vi "OAT Order Power Spectrum (1 Channel).vi"(0 "even-angle signal":cluster{"r0":dbl, "dr":dbl, "Y":dbl[]}={"r0"=0.0, "dr"=1.0, "Y"=[]} {"r0" format="%.2p"; "dr" format="%.2p"; "Y" format="%.2f"}, 1 "dB on? (T)":bool=TRUE, 5 "even-angle channel info":T1={"channel name"="", "description"="", " channel info"={"sensor sensitivity"=1000.0, "engineering units"=1, "dB reference"=1.0, "custom label"="EU", "weighting filter"=0, "pregain"=0.0}} {"channel info"."pregain" format="%.2f"; "channel info"."weighting filter" items=["Linear", "A-weighting", "B-weighting", "C-weighting", "ITU-R 468-4", "Dolby", "CCITT", "C-message", "Wb", "Wc", "Wd", "We", "Wf", "Wh", "Wj", "Wk", "Wm", "AES17 20 kHz lowpass", "AES17 40 kHz lowpass", "AES17 20 kHz highpass", "AES17 40 kHz highpass"]; "channel info"."dB reference" format="%^.1e"; "channel info"."engineering units" items=["custom..."=0, "V"=1, "A"=21, "C"=30, "pC"=31, "s"=32, "-"=29, "Pa"=2, "N"=20, "g"=3, "m/s^2"=4, "m/s"=5, "m"=6, "mm/s"=12, "mm"=13, "micron/s"=14, "micron"=15, "in/s^2"=7, "in/s"=8, "in"=9, "mil/s"=10, "mil"=11, "rad/s^2"=16, "rad/s"=17, "rad"=18, "deg/s^2"=26, "deg/s"=27, "deg"=28, "RPM"=22, "cycle/s^2"=23, "Hz"=24, "cycle"=25, "strain"=19]; "channel info"."sensor sensitivity" format="%#_5f"}, 7 "window":u32(ring)=1 items=["None"=0, "Hanning"=1, "Hamming"=2, "Blackman-Harris"=3, "Exact Blackman"=4, "Blackman"=5, "Flat Top"=6, "4 Term B-Harris"=7, "7 Term B-Harris"=8, "Low Sidelobe"=9, "Gaussian"=62], 9 "block size":i32=1024 min=2, 11 "error in (no error)":errorcluster, 12 "averaging parameters":T9={"averaging mode"=enum."No averaging", "weighting mode"=enum."Exponential", "number of averages"=10, "linear mode"=enum."One shot"} {"number of averages" min=1 step=1}, 13 "restart averaging? (F)":bool) -> (3 "new spectrum available?":bool, 4 "order power spectrum":T10={"order 0"=0.0, "delta order"=1.0, "magnitude"=[]} {"order 0" format="%.2p"; "delta order" format="%.2p"; "magnitude" format="%.2f"}, 6 "unit label":string, 8 "averages completed":dbl, 10 "spectrum info":T5={"channel name"="", "description"="", "x-axis units"=0, "spectral info"={"spectrum type"=enum."Power [Magnitude^2]", "linear/dB"=enum."linear", "window"=0, "window size"=0, "FFT size"=0}, "engineering units"=1, "custom label"="", "dB reference [EU]"=0.0, "peak units"=enum."rms", "weighting filter"=0, "spectral density?"=FALSE, "unit label"="", "spectrum skewed?"=FALSE, "complimentary spectrum units"=enum."none"} {"x-axis units" items=["Time (s)"=0, "Frequency-CB (Hz)"=1, "Frequency-CPB (Hz)"=1248, "Frequency-Arbitrary (Hz)"=2357, "Quefrency (s)"=2, "Revolutions (rev)"=3, "Order"=4, "Speed (RPM)"=11, "Speed (rad/s)"=21, "Index"=65535]; "weighting filter" items=["Linear", "A-weighting", "B-weighting", "C-weighting", "ITU-R 468-4", "Dolby", "CCITT", "C-message", "Wb", "Wc", "Wd", "We", "Wf", "Wh", "Wj", "Wk", "Wm", "AES17 20 kHz lowpass", "AES17 40 kHz lowpass", "AES17 20 kHz highpass", "AES17 40 kHz highpass"]; "dB reference [EU]" format="%.2f"; "engineering units" items=["custom..."=0, "V"=1, "A"=21, "C"=30, "pC"=31, "s"=32, "-"=29, "Pa"=2, "N"=20, "g"=3, "m/s^2"=4, "m/s"=5, "m"=6, "mm/s"=12, "mm"=13, "micron/s"=14, "micron"=15, "in/s^2"=7, "in/s"=8, "in"=9, "mil/s"=10, "mil"=11, "rad/s^2"=16, "rad/s"=17, "rad"=18, "deg/s^2"=26, "deg/s"=27, "deg"=28, "RPM"=22, "cycle/s^2"=23, "Hz"=24, "cycle"=25, "strain"=19]; "spectral info"."window" items=["None "=0, "Hanning"=1, "Hamming"=2, "Blackman-Harris"=3, "Exact Blackman"=4, "Blackman"=5, "Flat Top"=6, "4 Term B-Harris "=7, "7 Term B-Harris"=8, "Low Sidelobe"=9, "Force - Exponential"=10, "Gaussian"=62]}, 14 "averaging done?":bool, 15 "error out":errorcluster)   [LabVIEW 2017, in "SoundVib_OrderTracking.lvlib"]
doc: "Computes the order power spectrum of an even-angle signal. Wire data to the <B>even-angle signal</B> input to determine the polymorphic instance to use or manually select the instance."
uses:
  <vilib>/addons/Sound and Vibration/Order Analysis/Resample Order Tracking/SoundVib_OrderTracking.lvlib
  <vilib>/addons/_NISVFA/_Shared subVIs/Controls/svc_Spectrum Info.ctl
  <vilib>/addons/_NISVFA/_Shared subVIs/Controls/svc_X-Axis Units.ctl
  <vilib>/addons/_NISVFA/_Shared subVIs/Controls/svc_Spectrum Type.ctl
  <vilib>/addons/_NISVFA/_Shared subVIs/Controls/svc_Engineering Units Text Ring.ctl
  <vilib>/addons/_NISVFA/_Shared subVIs/Controls/svc_Weighting Filter Text Ring.ctl
  <vilib>/addons/_NISVFA/_Shared subVIs/Controls/svc_Complimentary Spectrum Units.ctl
  <vilib>/addons/_NISVFA/_Shared subVIs/Controls/svc_Resampled Channel Info.ctl
  <vilib>/addons/_NISVFA/_Shared subVIs/Controls/svc_Channel Info.ctl
  <vilib>/addons/Sound and Vibration/Order Analysis/Resample Order Tracking/SoundVib_Resampling.lvlib
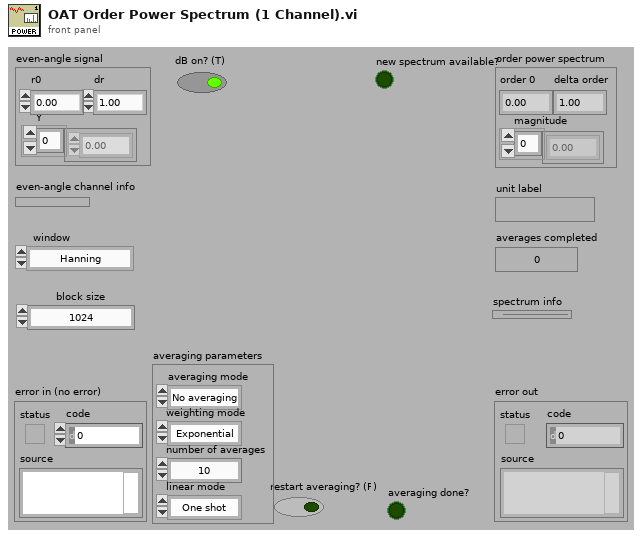
[diagram p1: front panel]
types:
  T1 = typedef "svc_Resampled Channel Info.ctl" = cluster{"channel name":string, "description":string, " channel info":T2}
  T2 = typedef "svc_Channel Info.ctl" = cluster{"sensor sensitivity":dbl, "engineering units":T3, "dB reference":dbl, "custom label":string, "weighting filter":T4, "pregain":dbl}
  T3 = typedef "svc_Engineering Units Text Ring.ctl" = u16
  T4 = typedef "svc_Weighting Filter Text Ring.ctl" = u16
  T5 = typedef "svc_Spectrum Info.ctl" = cluster{"channel name":string, "description":string, "x-axis units":T6, "spectral info":cluster{"spectrum type":T7, "linear/dB":enum16{"linear", "dB"}, "window":u16, "window size":i32, "FFT size":i32}, "engineering units":T3, "custom label":string, "dB reference [EU]":dbl, "peak units":enum16{"rms", "peak", "peak-peak"}, "weighting filter":T4, "spectral density?":bool, "unit label":string, "spectrum skewed?":bool, "complimentary spectrum units":T8}
  T6 = typedef "svc_X-Axis Units.ctl" = u16
  T7 = typedef "svc_Spectrum Type.ctl" = enum16{"FFT Spectrum [complex]", "Amplitude [Magnitude]", "Power [Magnitude^2]", "Cross Spectrum [complex]", "Frequency Response [Complex]"}
  T8 = typedef "svc_Complimentary Spectrum Units.ctl" = enum16{"none", "radians", "degrees", "cycles", "imaginary"}
  T9 = cluster{"averaging mode":enum16{"No averaging", "Vector averaging", "RMS averaging", "Peak hold"}, "weighting mode":enum16{"Linear", "Exponential"}, "number of averages":u32, "linear mode":enum16{"One shot", "Auto restart"}}
  T10 = cluster{"order 0":dbl, "delta order":dbl, "magnitude":dbl[]}
  T11 = cluster{"ignore dt":bool, "ignore t0 continuity":bool, "ignore array length":bool, "ignore channel info":bool, "ignore channel name":bool}
  T12 = cluster{"r0":dbl, "dr":dbl, "even angle signal":dbl[]}
  T13 = enum16{"Restart processing", "Continue processing", "Skip processing"}
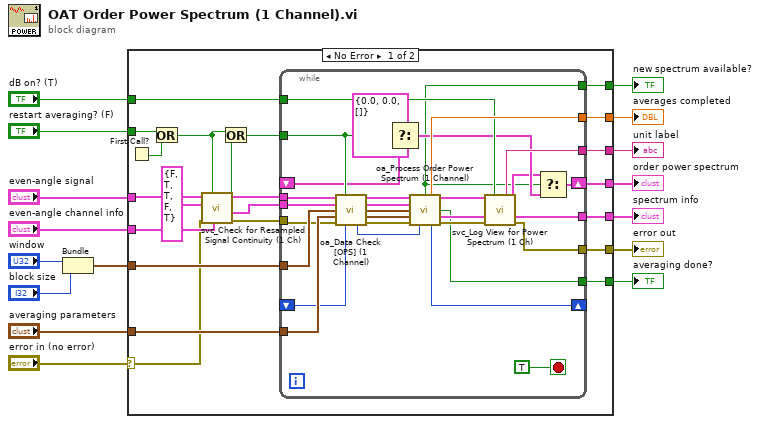
[diagram p0: block diagram]
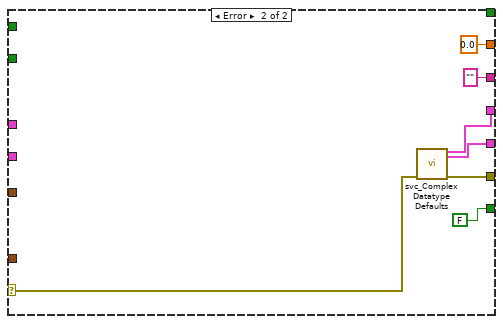
[diagram p2: hidden frame]
diagram:
  n1 = Bundle("window"="window", "block size"="block size") -> (w4:cluster{"window":u32, "block size":i32})  [unwired: 1 in]
  n2 = case shown="No Error" "error in (no error)" {
    selector: "error in (no error)" -> [w22 w74]
    tunnel: "even-angle signal" -> [w26 _]
    tunnel: "averaging parameters" -> [w38 _]
    tunnel: "restart averaging? (F)" -> [w29 _]
    tunnel: "even-angle channel info" -> [w24 _]
    tunnel: "dB on? (T)" -> [w37 _]
    tunnel: [w36 w74] -> w12
    tunnel: [w35 w70] -> w11
    tunnel: [w34 w69] -> w10
    tunnel: [w33 "" ("unit label")] -> w9
    tunnel: [w32 0.0 ("averages completed")] -> w8
    tunnel: [w31 FALSE ("averaging done")] -> w7
    tunnel: w4 -> [w30 _]
    tunnel: [w27 _] -> w1
    frame No Error {
      n3 = First Call?() -> (First Call?: T/F=w28:bool)
      n4 = Or(x=w29, y=w28) -> (x .or. y?=w20:bool)
      n5 = call <vilib>:"svc_Check for Resampled Signal Continuity (1 Ch).vi"("even angle channel info"=w24, "restart averaging (F)"=w20, "error in (no error)"=w22, "parameter controls"=T11 {"ignore dt"=FALSE, "ignore t0 continuity"=TRUE, "ignore array length"=TRUE, "ignore channel info"=FALSE, "ignore channel name"=TRUE}, "even angle signal"=w26) -> ("error out"=w21:errorcluster, "dup even angle channel info"=w23:T1, "waveform parameter changed"=w18:bool, "dup even angle signal"=w25:T12)  [unwired: 1 in, 2 out]
      n6 = Or(x=w20, y=w18) -> (x .or. y?=w19:bool)
      n7 = while {
        tunnel: w25 -> [w68]
        tunnel: w38 -> [w67]
        tunnel: w19 -> [w47]
        tunnel: w23 -> [w50]
        tunnel: w37 -> [w48]
        tunnel: [w58] -> w36
        tunnel: [w57] -> w35
        tunnel: [w56] -> w33
        tunnel: [w55] -> w32
        tunnel: [w41] -> w31
        shift-right: [w52] -> _
        shift-left: _ -> [w53]
        tunnel: w30 -> [w51]
        tunnel: [w40] -> w27
        shift-right: [w44] -> w34
        shift-left: _ -> [w46]
        tunnel: w21 -> [w39]
        stop <- TRUE stop-if-true
        n8 = call <vilib>:"oa_Data Check [OPS] (1 Channel).vi"("resampled signal"=w68, "restart averaging (F)"=w47, "resampled channel info"=w50, "spectrum settings"=w51, "averaging parameters"=w67, "error in (no error)"=w39, "processing control in"=w53) -> ("dup resampled signal"=w62:cluster{"r0":dbl, "dr":dbl, "Y":dbl[]}, "dup resampled channel info"=w49:T1, "dup spectrum settings"=w63:cluster{"window type":u32, "block size":i32}, "dup averaging parameters"=w64:T9, "processing control out"=w66:T13, "error out"=w65:errorcluster)  [unwired: 3 in]
        n9 = Select(t=cluster{"f0":dbl, "df":dbl, "magnitude":dbl[]} {"f0"=0.0, "df"=0.0, "magnitude"=[]}, s=w47, f=w46) -> (s? t:f=w43:cluster{"f0":dbl, "df":dbl, "magnitude":dbl[]})
        n10 = call <vilib>:"oa_Process Order Power Spectrum (1 Channel).vi"("resampled signal"=w62, "resampled channel info"=w49, "spectrum settings"=w63, "averaging parameters"=w64, "error in"=w65, "processing control in"=w66) -> ("new spectrum available?"=w40:bool, "averages completed"=w55:dbl, "order spectrum"=w61:T10, "averaging done"=w41:bool, "spectrum info"=w60:T5, "processing control out"=w52:T13, "error out"=w59:errorcluster)  [unwired: 3 in]
        n11 = call <vilib>:"svc_Log View for Power Spectrum (1 Ch).vi"("power spectrum [dB EU]"=w61, "dB On (T)"=w48, "spectrum info"=w60, "error in (no error)"=w59) -> ("unit label"=w56:string, "power spectrum [dB EU]"=w42:cluster{"f0":dbl, "df":dbl, "magnitude":dbl[]}, "spectrum info out"=w57:T5, "error out"=w58:errorcluster)  [unwired: 8 in]
        n12 = Select(t=w42, s=w40, f=w43) -> (s? t:f=w44:cluster{"f0":dbl, "df":dbl, "magnitude":dbl[]})
      }
    }
    frame Error {
      n13 = call <vilib>:"svc_Complex Datatype Defaults.vi"() -> ("empty spectrum"=w69:cluster{"f0":dbl, "df":dbl, "magnitude":dbl[]}, "dead spectrum info"=w70:T5)  [unwired: 11 in, 7 out]
    }
  }
  "order power spectrum" <- w10
  "unit label" <- w9
  "error out" <- w12
  "averaging done?" <- w7
  "averages completed" <- w8
  "spectrum info" <- w11
  "new spectrum available?" <- w1
